vi "VisitLVClusterType.vi"(8 "error in (no error)":errorcluster, 10 "LVClusterType":refnum<class "LVClusterType.lvclass">, 11 "GetTypeAttributesVisitor in":refnum<class "GetTypeAttributesVisitor.lvclass">) -> (0 "error out":errorcluster, 3 "GetTypeAttributesVisitor out":refnum<class "GetTypeAttributesVisitor.lvclass">)   [LabVIEW 2020, in "Web Service Description.lvlib" / "GetTypeAttributesVisitor.lvclass"]
uses:
  <vilib>/AppBuilder/Engine/WebServiceDescription/GetTypeAttributesVisitor/GetTypeAttributesVisitor.lvclass
  <vilib>/AppBuilder/Engine/WebServiceDescription/LVDataTypes/LVClusterType/LVClusterType.lvclass
  e:/builds/penguin/labview/branches/2020/dev/dist/vi.lib/AppBuilder/Engine/WebServiceDescription/LVDataTypes/LVType/LVType.lvclass
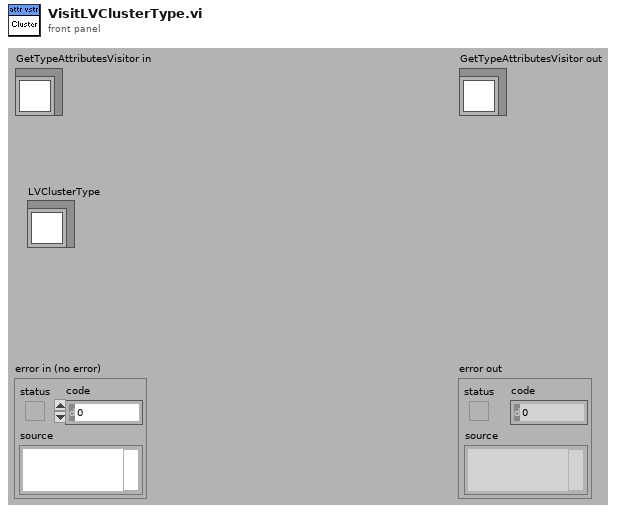
[diagram p1: front panel]
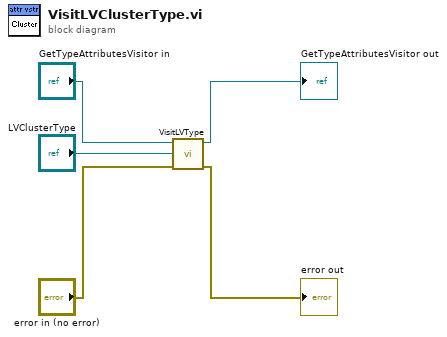
[diagram p0: block diagram]
diagram:
  n1 = call-dynamic "VisitLVType.vi"("error in (no error)"="error in (no error)", "LVType"="LVClusterType", "GetTypeAttributesVisitor in"="GetTypeAttributesVisitor in") -> ("error out"=→"error out":errorcluster, "GetTypeAttributesVisitor out"=→"GetTypeAttributesVisitor out":refnum<class "GetTypeAttributesVisitor.lvclass">)  [unwired: 7 out]
